vi "AsynchronousData_Lab9.vi"() -> ()   [LabVIEW 2016]
panel:
  out "Master Boolean":bool
  in  "?":bool
  out "?":dbl(slide) scale=0.0..1.0
  out "?":dbl(slide) scale=0.0..1.0
  in  "?":bool
  out "Vertical":dbl
  out "Horizontal":dbl
  in  "?":bool
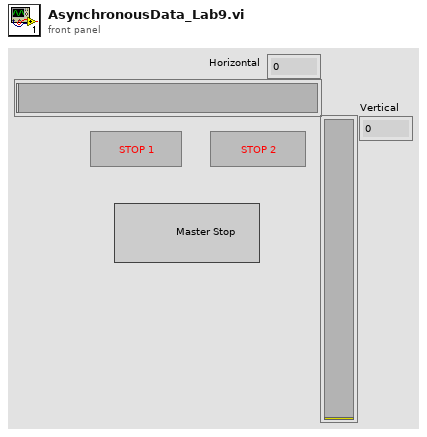
[diagram p1: front panel]
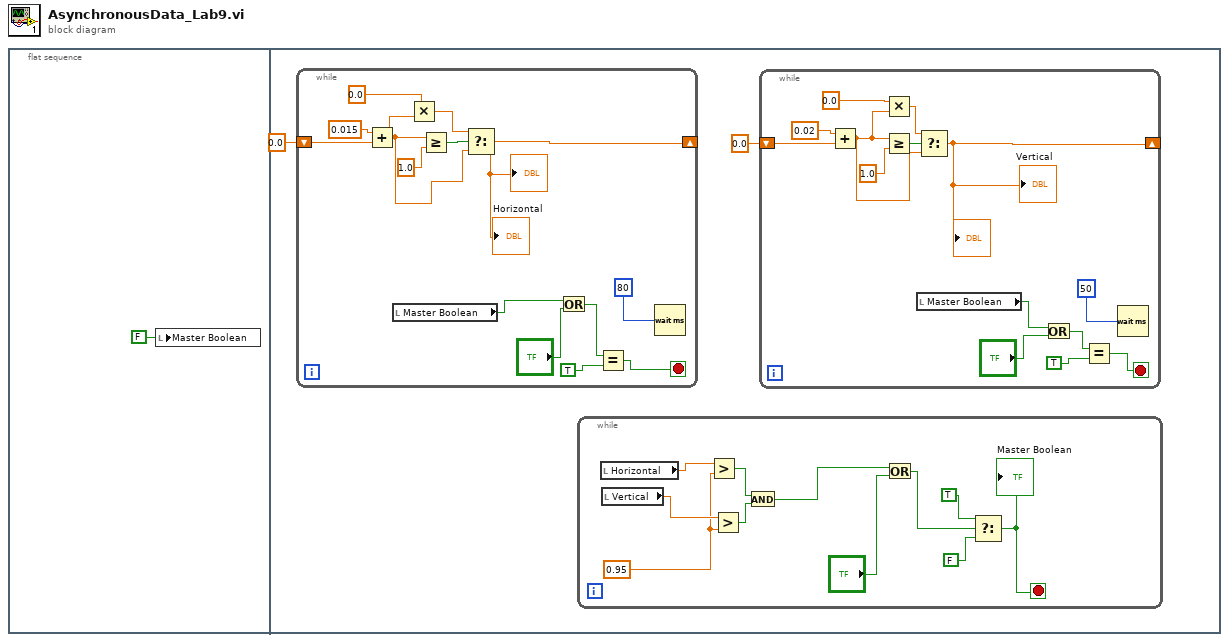
[diagram p0: block diagram]
diagram:
  n1 = flat-sequence {
    frame #0 {
      n2 = local write "Master Boolean"(FALSE ("Master Boolean")) -> ()
    }
    frame #1 {
      n3 = while {
        shift-right: [w35] -> _
        shift-left: 0.0 -> [w42]
        stop <- w29 stop-if-true
        n4 = Add(x=0.015, y=w42) -> (x+y=w32:dbl)
        n5 = local read "Master Boolean"() -> (w33:bool)
        n6 = Multiply(x=0.0, y=w32) -> (x*y=w37:dbl)
        n7 = Greater Or Equal?(x=w32, y=1.0) -> (x >= y?=w39:bool)
        n8 = Select(t=w37, s=w39, f=w32) -> (s? t:f=w35:dbl)
        "Horizontal" <- w35
        "?" <- w35
        n9 = Or(x=w33, y="?") -> (x .or. y?=w30:bool)
        n10 = Equal?(x=w30, y=TRUE) -> (x = y?=w29:bool)
        n11 = Wait (ms)(milliseconds to wait=u32 80) -> ()  [unwired: 1 out]
      }
      n12 = while {
        stop <- w10 stop-if-true
        w7 = 0.95
        n13 = local read "Horizontal"() -> (w9:dbl)
        n14 = local read "Vertical"() -> (w8:dbl)
        n15 = Greater?(x=w9, y=w7) -> (0:w6:bool)
        n16 = Greater?(x=w8, y=w7) -> (0:w5:bool)
        n17 = And(x=w6, y=w5) -> (x .and. y?=w4:bool)
        n18 = Or(x=w4, y="?") -> (x .or. y?=w12:bool)
        n19 = Select(t=TRUE, s=w12, f=FALSE) -> (s? t:f=w10:bool)
        "Master Boolean" <- w10
      }
      n20 = while {
        shift-right: [w21] -> _
        shift-left: 0.0 -> [w28]
        stop <- w15 stop-if-true
        n21 = Add(x=0.02, y=w28) -> (x+y=w18:dbl)
        n22 = Multiply(x=0.0, y=w18) -> (x*y=w23:dbl)
        n23 = Greater Or Equal?(x=w18, y=1.0) -> (x >= y?=w25:bool)
        n24 = local read "Master Boolean"() -> (w19:bool)
        n25 = Select(t=w23, s=w25, f=w18) -> (s? t:f=w21:dbl)
        "Vertical" <- w21
        "?" <- w21
        n26 = Or(x=w19, y="?") -> (x .or. y?=w17:bool)
        n27 = Equal?(x=w17, y=TRUE) -> (x = y?=w15:bool)
        n28 = Wait (ms)(milliseconds to wait=u32 50) -> ()  [unwired: 1 out]
      }
    }
  }
